vi "Secure Client Example.vi"() -> ()   [LabVIEW 2020]
doc: "A simple WebSockets client example using Secure WebSockets (wss://)."
uses:
  Secure WebSocket Client/Secure WebSockets Client.lvclass
panel:
  in  "Client Certificate Path":path
  in  "Send":bool
  out "Read Text":string
  in  "Write Text":string="Hello World!"
  in  "WebSocket URL":string="wss://locahost:7123"
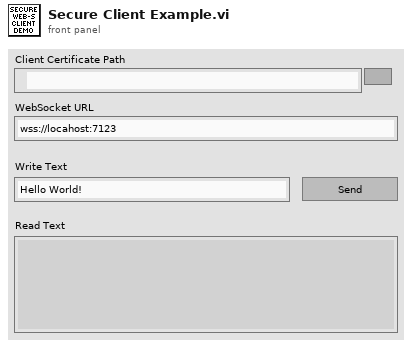
[diagram p1: front panel]
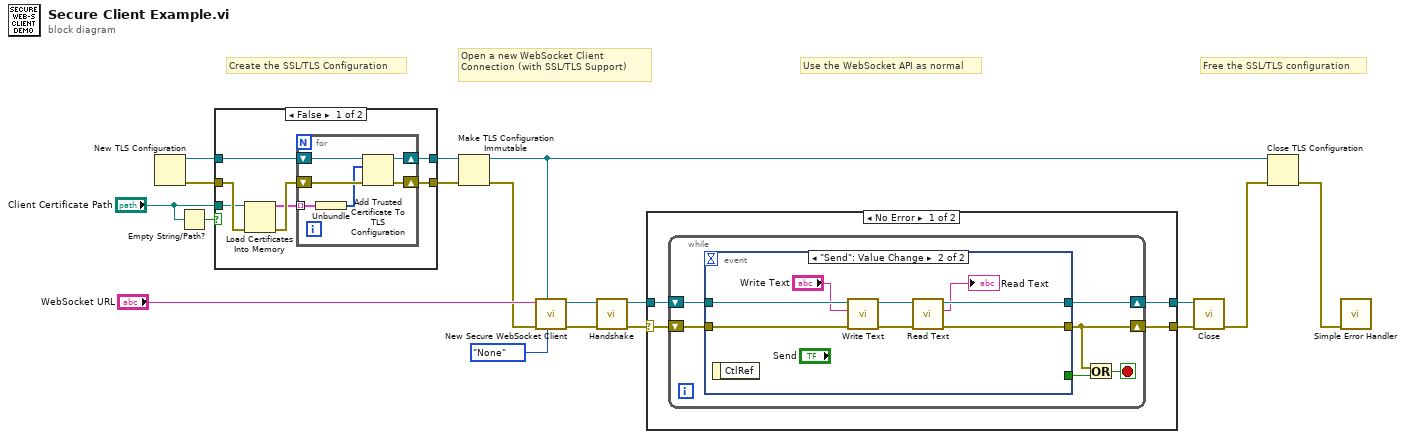
[diagram p0: block diagram]
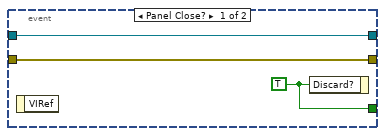
[diagram p3: hidden frame]
diagram:
  # "Free the SSL/TLS configuration"
  # "Use the WebSocket API as normal"
  # "Open a new WebSocket Client Connection (with SSL/TLS Support)"
  # "Create the SSL/TLS Configuration"
  n1 = New TLS Configuration() -> (0:w1:errorcluster, 3:w2:refnum<k36>)  [unwired: 2 in]
  n2 = Empty String/Path?(string/path="Client Certificate Path") -> (empty?=w5:bool)
  n3 = case shown="False" w5 {
    tunnel: w2 -> [w25 w33]
    tunnel: w1 -> [w24 w32]
    tunnel: [w21 w32] -> w3
    tunnel: [w20 w33] -> w4
    tunnel: "Client Certificate Path" -> [w19 _]
    frame False {
      n4 = Load Certificates Into Memory(8:w24, 11:w19) -> (0:w23:errorcluster, 3:w22:cluster{"certificate":u8[]}[])  [unwired: 1 in]
      n5 = for {
        shift-right: [w29] -> w20
        shift-left: w25 -> [w30]
        shift-right: [w28] -> w21
        shift-left: w23 -> [w31]
        tunnel: w22 -> [w27] mode=indexing
        n6 = Unbundle(w27) -> ("certificate"=w26:u8[])
        n7 = Add Trusted Certificate To TLS Configuration(8:w31, 10:w26, 11:w30) -> (0:w28:errorcluster, 3:w29:refnum<k36>)  [unwired: 1 in]
      }
    }
    frame True {
    }
  }
  n8 = Make TLS Configuration Immutable(8:w3, 11:w4) -> (0:w9:errorcluster, 3:w8:refnum<k36>)
  n9 = call "New Secure WebSocket Client.vi"("server certificate validation"=enum32{"Any Trusted CA", "None"}."None", "immutable TLS Configuration"=w8, "error in (no error)"=w9, "WebSocket URL"="WebSocket URL") -> ("error out"=w16:errorcluster, "Secure WebSockets Client out"=w17:refnum<class "Secure WebSockets Client.lvclass">)  [unwired: 6 in]
  n10 = call-dynamic "Handshake.vi"("error in (no error)"=w16, "WebSocket Client in"=w17) -> ("error out"=w15:errorcluster, "WebSocket Client out"=w14:refnum<class "Secure WebSockets Client.lvclass">)  [unwired: 8 in]
  n11 = case shown="No Error" w15 {
    selector: w15 -> [w37 w56]
    tunnel: w14 -> [w36 w55]
    tunnel: [w35 w55] -> w13
    tunnel: [w34 w56] -> w12
    frame No Error {
      n12 = while {
        shift-right: [w41] -> w35
        shift-left: w36 -> [w42]
        shift-right: [w39] -> w34
        shift-left: w37 -> [w43]
        stop <- w38 stop-if-true
        n13 = event shown="[1] \"Send\": Value Change" {
          selector: _ -> [_ _]
          dyn-events: _ -> [_ _]
          timeout: _ -> [_ _]
          tunnel: [w46 _] -> w40
          tunnel: w43 -> [w44 w53]
          tunnel: w42 -> [w45 w52]
          tunnel: [w45 w50] -> w41
          tunnel: [w44 w49] -> w39
          event Panel Close? {
            w46 = TRUE ("Discard?")
            n14 = event-data() -> ()  [unwired: 1 in, 1 out]
            n15 = event-data("Discard?"=w46) -> ()  [unwired: 1 in, 1 out]
          }
          event "Send": Value Change {
            n16 = event-data() -> ()  [unwired: 1 in, 1 out]
            n17 = call-dynamic "Write Text.vi"("error in (no error)"=w53, "String Data"="Write Text", "WebSocket in"=w52) -> ("error out"=w54:errorcluster, "WebSocket out"=w51:refnum<class "Secure WebSockets Client.lvclass">)  [unwired: 7 in]
            n18 = call-dynamic "Read Text.vi"("error in (no error)"=w54, "WebSocket in"=w51) -> ("error out"=w49:errorcluster, "Data"=→"Read Text":string, "WebSocket out"=w50:refnum<class "Secure WebSockets Client.lvclass">)  [unwired: 7 in]
          }
        }
        n19 = Or(x=w39, y=w40) -> (x .or. y?=w38:bool)
      }
    }
    frame Error {
    }
  }
  n20 = call-dynamic "Close.vi"("error in (no error)"=w12, "WebSocket in"=w13) -> ("error out"=w11:errorcluster)  [unwired: 9 in]
  n21 = Close TLS Configuration(8:w11, 11:w8) -> (0:w10:errorcluster)
  n22 = call <vilib>:"Simple Error Handler.vi"("error in (no error)"=w10) -> ()  [unwired: 4 in, 5 out]
